vi "Show Sequence.vi"(0 "object in":refnum<class "Hamamatsu.lvclass">, 2 "Enum":enum16{"Get Path", "RunAsync"}(ring)=enum."RunAsync", 5 "error in (no error)":errorcluster) -> (14 "object out":refnum<class "Hamamatsu.lvclass">, 16 "path":path, 19 "error out":errorcluster)   [LabVIEW 2021, in "Hamamatsu.lvclass"]
uses:
  Hamamatsu.lvclass
  Hamamatsu.lvclass/Hamamatsu.ctl
panel:
  in  "Numeric":u16
  out "Image":T1(plugin-control)
  in  "Close":bool
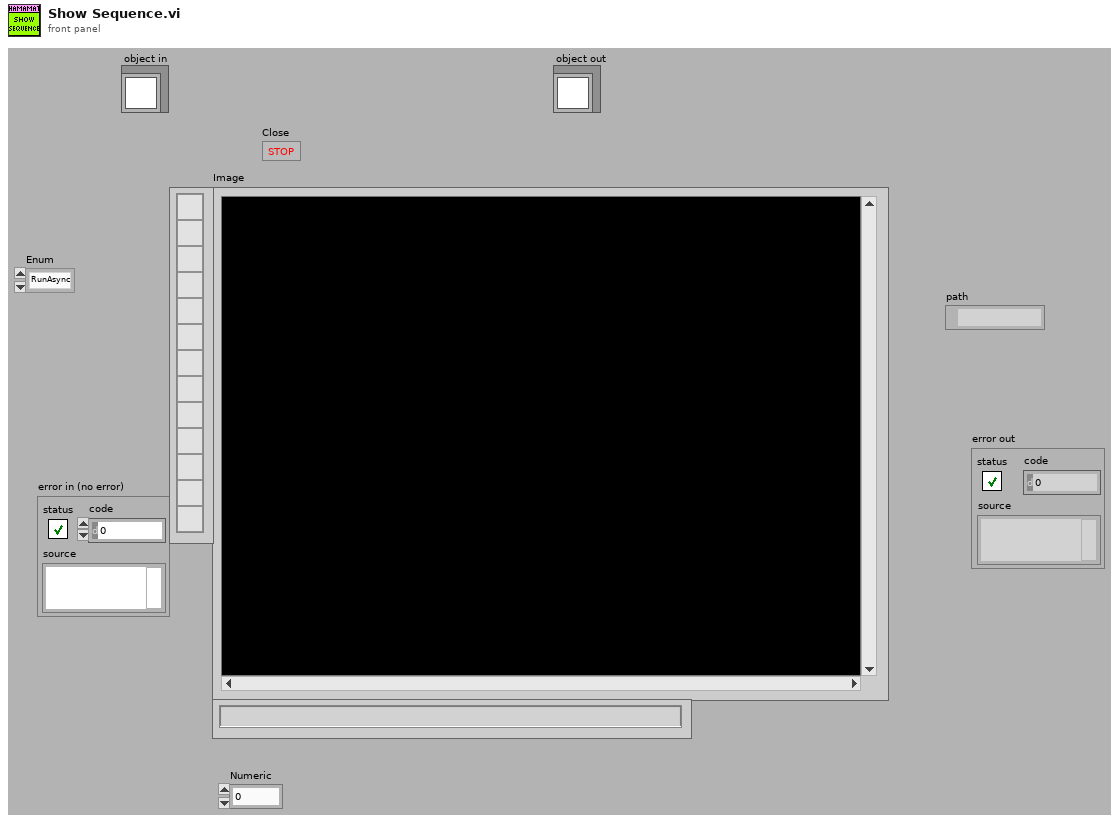
[diagram p1: front panel]
types:
  T1 = typedef "IMAQ Image.ctl" = refnum<image>
  T2 = typedef "Image Type" = u32
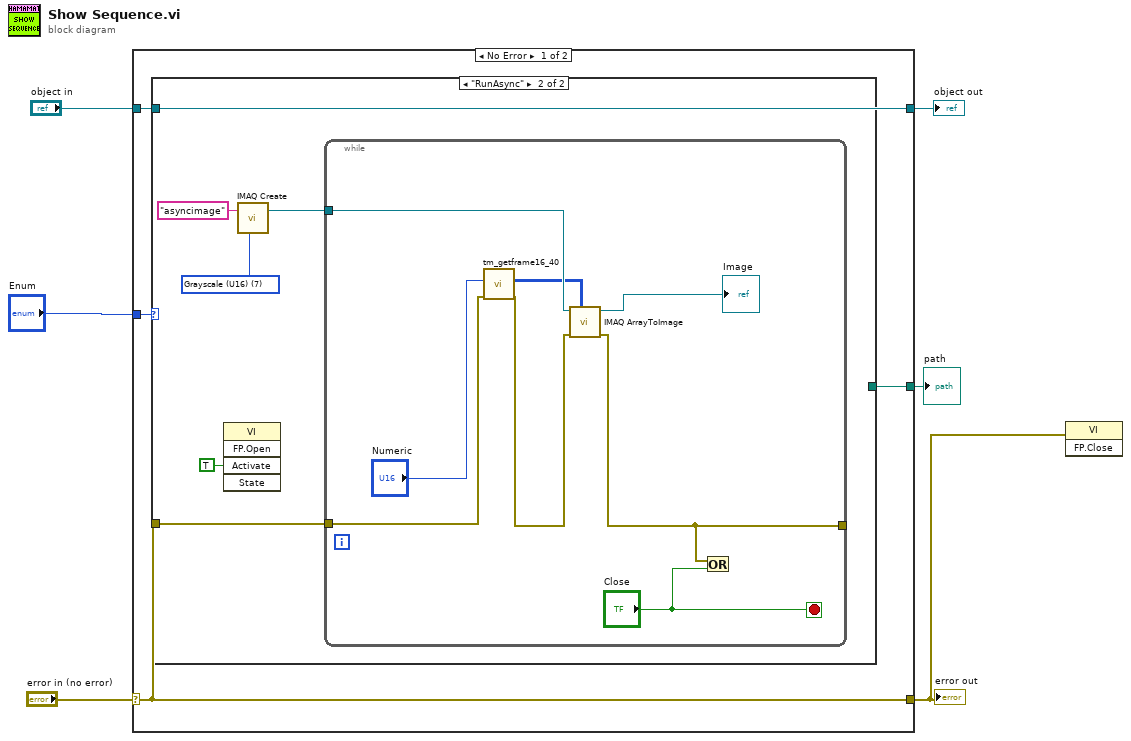
[diagram p0: block diagram]
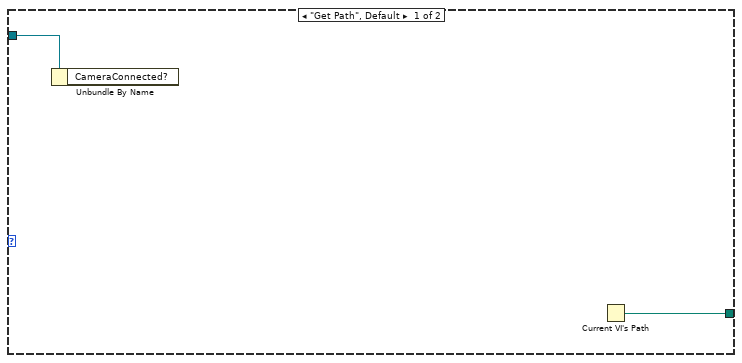
[diagram p2: hidden frame]
diagram:
  n1 = case shown="No Error" "error in (no error)" {
    selector: "error in (no error)" -> [w7 w27]
    tunnel: [w7 w27] -> w1
    tunnel: [w10 w26] -> w4
    tunnel: "object in" -> [w10 w26]
    tunnel: [w9 _] -> w3
    tunnel: "Enum" -> [w8 _]
    frame No Error {
      n2 = case shown="\"RunAsync\"" w8 {
        tunnel: w10 -> [w12 _]
        tunnel: [w11 _] -> w9
        tunnel: w7 -> [_ w16]
        frame "Get Path", Default {
          n3 = Unbundle By Name(w12) -> ()  [unwired: 1 out]
          n4 = Current VI's Path() -> (path=w11:path)
        }
        frame "RunAsync" {
          w14 = T2 7 items=["Grayscale (U8)", "Grayscale (I16)", "Grayscale (SGL)", "Complex (CSG)", "RGB (U32)", "HSL (U32)", "RGB (U64)", "Grayscale (U16)"] ("Image Type")
          n5 = invoke class="VI" method="FP.Open"("Activate"=TRUE ("Activate?")) -> ()  [unwired: 4 in, 5 out]
          n6 = call "IMAQ Create"("Image Name"="asyncimage", "Image Type"=w14) -> ("New Image"=w15:T1)  [unwired: 3 in, 1 out]
          n7 = while {
            tunnel: w16 -> [w25]
            tunnel: w15 -> [w23]
            tunnel: [w19] -> _
            stop <- "Close" stop-if-true
            n8 = call <userlib>:"tm_getframe16_40.vi"("error in (no error)"=w25, "Frame Index"="Numeric") -> ("error out"=w20:errorcluster, "Data"=w18:u16[][])  [unwired: 6 in, 2 out]
            n9 = call "IMAQ ArrayToImage"("Image Pixels (U16)"=w18, "error in (no error)"=w20, "Image"=w23) -> ("error out"=w19:errorcluster, "Image Out"=→"Image":T1)  [unwired: 7 in]
            n10 = Or(x=w19, y="Close") -> ()  [unwired: 1 out]
          }
        }
      }
    }
    frame Error {
    }
  }
  "error out" <- w1
  "object out" <- w4
  "path" <- w3
  n11 = invoke class="VI" method="FP.Close"(error in=w1) -> ()  [unwired: 2 in, 3 out]
